vi "Insight_Initiate_Measurements.vi"(7 "Channel (2)":enum16{"1", "2", "3"}(ring)=enum."2", 8 "error in (no error)":errorcluster, 9 "Timeout, sec":u32=3, 10 "Continuous (On)":enum16{"Off", "On"}(ring)=enum."On", 11 "telnet connection":T1) -> (0 "error out":errorcluster, 1 "response data":string, 3 "telnet  connection out":T1)   [LabVIEW 2011]
doc: "Insight Photonic Solutions\n\nThis VI initiates measurements by the laser. Measurements made be made simultaneously on up to 3 channels (default: channel 2). Measurements may be performed either as a single acquisition or continuously (Default: continuous).\n\nver 1.0 - original release, 1/30/2013. Channel selection option and Continuous On/Off options are disabled. The measurement is always operating on Channel 2 for the first implementation in the laser."
uses:
  Telnet Session.ctl
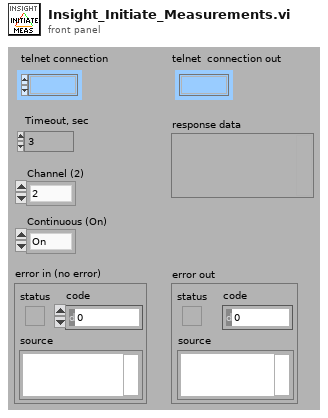
[diagram p1: front panel]
types:
  T1 = typedef "Telnet Session.ctl" = refnum<k1>
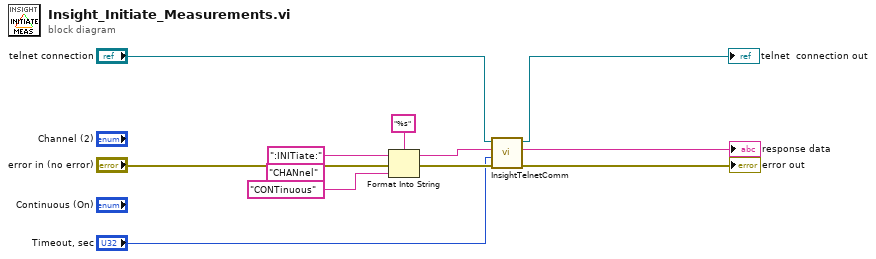
[diagram p0: block diagram]
diagram:
  (unwired) "CHANnel"
  n1 = Format Into String(format string="%s", initial string=":INITiate:" ("String"), error in="error in (no error)", "CONTinuous") -> (resulting string=w5:string, error out=w3:errorcluster)
  n2 = call "InsightTelnetComm.vi"("error in"=w3, "Timeout, sec"="Timeout, sec", "write buffer (\"\")"=w5, "telnet connection"="telnet connection") -> ("error out"=→"error out":errorcluster, "response data"=→"response data":string, "telnet  connection out"=→"telnet  connection out":T1)  [unwired: 3 in]
